vi "Recursively Create Menus.vi"(5 "Parent":refnum<vi>, 7 "菜单标识符":string, 8 "错误输入（无错误）":errorcluster, 9 "项标识符":string, 10 "项名称":string, 11 "菜单引用 in":refnum<k9>) -> (0 "错误输出":errorcluster, 2 "Menu Items To Add":T1[](array[typedef]) caption="待添加菜单项", 3 "菜单引用 out":refnum<k9>)   [LabVIEW 2020]
uses:
  <resource>/plugins/PopupMenus/support/Shortcut Menu Item Definition.ctl
  <resource>/plugins/PopupMenus/support/Transaction Control.ctl
  <resource>/plugins/PopupMenus/support/Position In Menu.ctl
  <resource>/plugins/PopupMenus/support/Relative Position.ctl
  <resource>/plugins/PopupMenus/support/Checkmark Status.ctl
  <resource>/plugins/PopupMenus/support/Enabled Menu Item Status.ctl
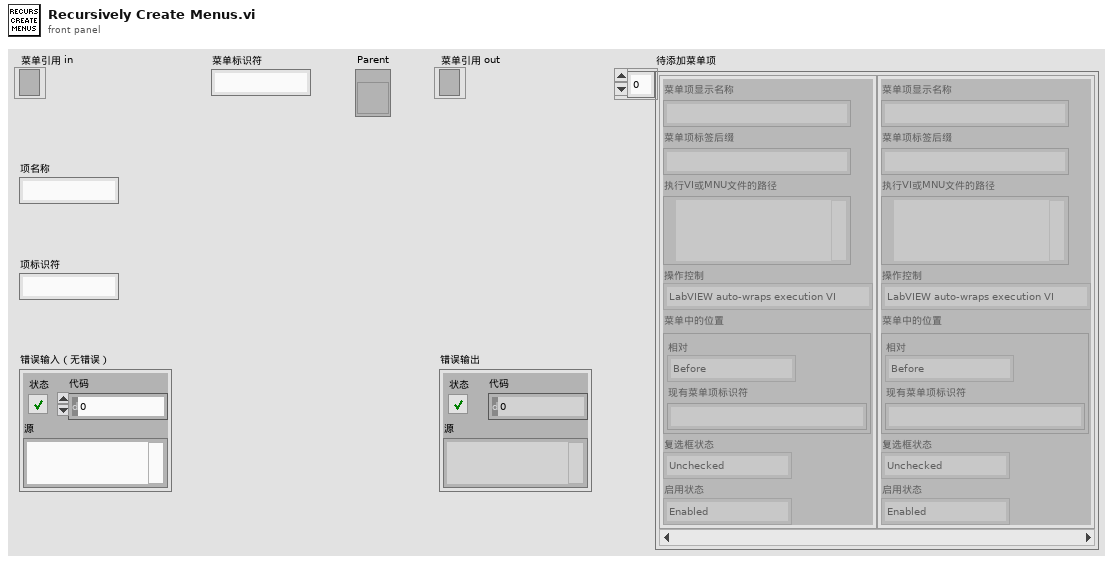
[diagram p1: front panel]
types:
  T1 = typedef "Shortcut Menu Item Definition.ctl" = cluster{"Menu Item Display Name":string, "Menu Item Tag Suffix":string, "Path To Execution VI or MNU":path, "Transaction Control":T2, "Position In Menu":T3, "Checkmark Status":T5, "Enabled Status":T6}
  T2 = typedef "Transaction Control.ctl" = enum8{"LabVIEW auto-wraps execution VI", "Execution VI will define if needed"}
  T3 = typedef "Position In Menu.ctl" = cluster{"Relative":T4, "Existing Item Tag":string}
  T4 = typedef "Relative Position.ctl" = enum8{"Before", "Instead of", "After", "Into Submenu"}
  T5 = typedef "Checkmark Status.ctl" = enum8{"Unchecked", "Checked"}
  T6 = typedef "Enabled Menu Item Status.ctl" = enum8{"Enabled", "Disabled"}
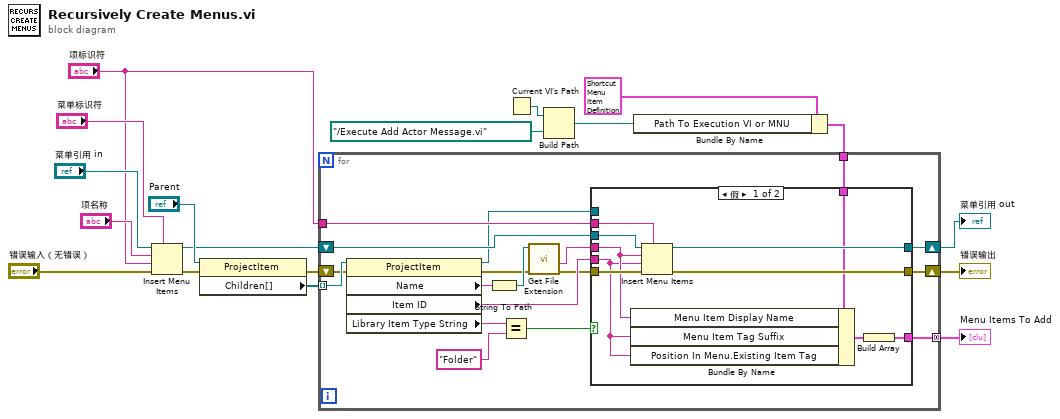
[diagram p0: block diagram]
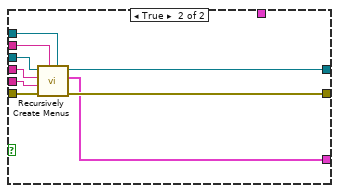
[diagram p2: hidden frame]
diagram:
  n1 = Insert Menu Items(5:"菜单标识符", 6:"错误输入（无错误）", 7:"项标识符", 8:"项名称", 9:"菜单引用 in") -> (0:w9:errorcluster, 3:w13:refnum<k9>)  [unwired: 1 in, 1 out]
  n2 = property class="ProjectItem"(reference="Parent", error in=w9) -> (error out=w8:errorcluster, "Children[]"=w17:refnum<vi>[])  [unwired: 1 out]
  n3 = Current VI's Path() -> (path=w2:path)
  n4 = Build Path(base path=w2, name or relative path=path "../Execute Add Actor Message.vi" ("execute path")) -> (appended path=w1:path)
  n5 = Bundle By Name(cluster=T1 {"Menu Item Display Name"="", "Menu Item Tag Suffix"="", "Path To Execution VI or MNU"=path "", "Transaction Control"=enum."LabVIEW auto-wraps execution VI", "Position In Menu"={"Relative"=enum."Instead of", "Existing Item Tag"=""}, "Checkmark Status"=enum."Unchecked", "Enabled Status"=enum."Enabled"} ("Cluster"), "Path To Execution VI or MNU"=w1) -> (w4:T1)
  n6 = for {
    tunnel: w17 -> [w36] mode=indexing
    tunnel: "项标识符" -> [w31]
    shift-right: [w28] -> w11
    shift-left: w13 -> [w33]
    shift-right: [w29] -> w7
    shift-left: w8 -> [w30]
    tunnel: [w25] -> w6 mode=concatenating
    tunnel: w4 -> [w19]
    n7 = property class="ProjectItem"(reference=w36, error in=w30) -> (reference out=w26:refnum<vi>, error out=w20:errorcluster, "Name"=w23:string, "Item ID"=w32:string, "Library Item Type String"=w35:string)
    n8 = String To Path(string=w23) -> (path=w24:path)
    n9 = Equal?(x=w35, y="Folder") -> (x = y?=w27:bool)
    n10 = call <vilib>:"Get File Extension.vi"("error in (no error)"=w20, "file"=w24) -> ("error out"=w21:errorcluster, "filename without extension"=w22:string)  [unwired: 5 in, 3 out]
    n11 = case shown="假" w27 {
      tunnel: w33 -> [w46 w52]
      tunnel: w22 -> [w41 w48]
      tunnel: w32 -> [w40 w49]
      tunnel: w31 -> [w45 w50]
      tunnel: w21 -> [w44 w55]
      tunnel: [w43 w54] -> w29
      tunnel: [w42 w53] -> w28
      tunnel: w26 -> [_ w51]
      tunnel: [w38 w47] -> w25
      tunnel: w19 -> [w37 _]
      frame False {
        n12 = Bundle By Name(cluster=w37, "Menu Item Display Name"=w41, "Menu Item Tag Suffix"=w40, "Position In Menu.Existing Item Tag"=w40) -> (w39:T1)
        n13 = Insert Menu Items(5:w45, 6:w44, 7:w40, 8:w41, 9:w46) -> (0:w43:errorcluster, 3:w42:refnum<k9>)  [unwired: 1 in, 1 out]
        n14 = Build Array(w39) -> (w38:T1[])
      }
      frame True {
        n15 = call "Recursively Create Menus.vi"("Parent"=w51, "菜单标识符"=w50, "错误输入（无错误）"=w55, "项标识符"=w49, "项名称"=w48, "菜单引用 in"=w52) -> ("错误输出"=w54:errorcluster, "Menu Items To Add"=w47:T1[], "菜单引用 out"=w53:refnum<k9>)  [unwired: 3 in]
      }
    }
  }
  "菜单引用 out" <- w11
  "错误输出" <- w7
  "Menu Items To Add" <- w6
